vi "Client.vi"() -> ()   [LabVIEW 2011]
uses:
  Singleton/Singleton.lvclass
panel:
  in  "Stop":bool
  out "Boolean":bool
  in  "Toggle":bool
  # "The DVR becomes invalid\n when its originator\n leaves memory."
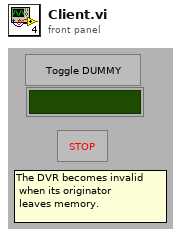
[diagram p1: front panel]
types:
  T1 = typedef "Singleton.lvclass/Instance handle.ctl" = refnum<data-value>
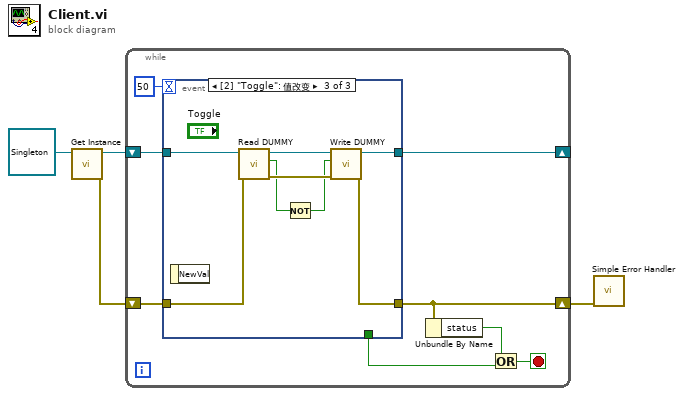
[diagram p0: block diagram]
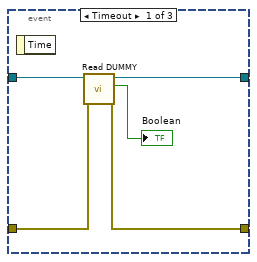
[diagram p2: hidden frame]
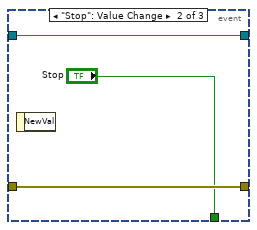
[diagram p3: hidden frame]
diagram:
  n1 = call "Get Instance.vi"("Singleton"=refnum<class "Singleton.lvclass"> refnum ("Singleton Abstract.lvclass")) -> ("error out"=w2:errorcluster, "Instance Handle"=w3:T1)  [unwired: 9 in]
  n2 = while {
    shift-right: [w11] -> _
    shift-left: w3 -> [w12]
    shift-right: [w8] -> w1
    shift-left: w2 -> [w10]
    stop <- w6 stop-if-true
    n3 = event shown="[2] \"Toggle\": 值改变" {
      selector: _ -> [_ _ _]
      dyn-events: _ -> [_ _ _]
      timeout: 50 -> [_ _ _]
      tunnel: w12 -> [w17 w20 w28]
      tunnel: [w16 w20 w26] -> w11
      tunnel: w10 -> [w14 w19 w24]
      tunnel: [w13 w19 w23] -> w8
      tunnel: [_ "Stop" _] -> w5
      event Timeout {
        n4 = event-data() -> ()  [unwired: 1 in, 1 out]
        n5 = call "Read DUMMY.vi"("error in (no error)"=w14, "Instance Handle"=w17) -> ("error out"=w13:errorcluster, "DUMMY"=→"Boolean":bool, "Session Handle Out"=w16:T1)  [unwired: 7 in]
      }
      event "Stop": Value Change {
        n6 = event-data() -> ()  [unwired: 1 in, 1 out]
      }
      event "Toggle": Value Change {
        n7 = event-data() -> ()  [unwired: 1 in, 1 out]
        n8 = call "Read DUMMY.vi"("error in (no error)"=w24, "Instance Handle"=w28) -> ("error out"=w25:errorcluster, "DUMMY"=w22:bool, "Session Handle Out"=w27:T1)  [unwired: 7 in]
        n9 = Not(x=w22) -> (.not. x?=w21:bool)
        n10 = call "Write DUMMY.vi"("error in (no error)"=w25, "DUMMY"=w21, "Instance Handle"=w27) -> ("error out"=w23:errorcluster, "Session Handle Out"=w26:T1)  [unwired: 7 in]
      }
    }
    n11 = Unbundle By Name(w8) -> ("status"=w7:bool)
    n12 = Or(x=w7, y=w5) -> (x .or. y?=w6:bool)
  }
  n13 = call <vilib>:"Simple Error Handler.vi"("error in (no error)"=w1) -> ()  [unwired: 4 in, 5 out]
